vi "Construct.vi"(1 "Color":u32(colorbox), 2 "Height":i16, 3 "Width":i16) -> (0 "RectangleShape out":refnum<class "RectangleShape.lvclass">)   [LabVIEW 2022 SP3, in "RectangleShape.lvclass"]
uses:
  RectangleShape.lvclass
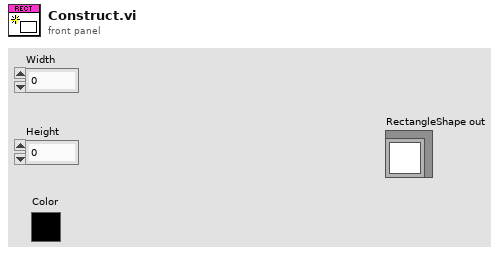
[diagram p1: front panel]
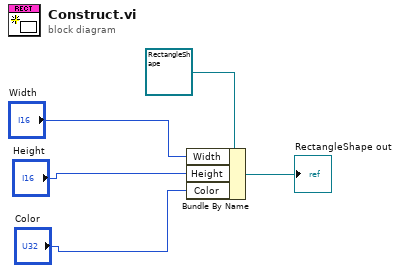
[diagram p0: block diagram]
diagram:
  n1 = Bundle By Name(cluster=refnum<class "RectangleShape.lvclass"> refnum ("RectangleShape.lvclass"), "Width"="Width", "Height"="Height", "Color"="Color") -> (→"RectangleShape out":refnum<class "RectangleShape.lvclass">)
